vi "reportError.vi"(8 "ErrorIn":errorcluster, 10 "ErrorType":T1, 11 "QueuesIn":T2) -> (0 "ErrorOut":errorcluster, 3 "QueuesOut":T2)   [LabVIEW 2019]
uses:
  utilities/Queues.ctl
  UIVIs/UIInput.ctl
  UIVIs/UIOutput.ctl
  UIVIs/AccelerationDataFrames.ctl
  communicateWebServicesVIs/WebServicesData.ctl
  ErrorType.ctl
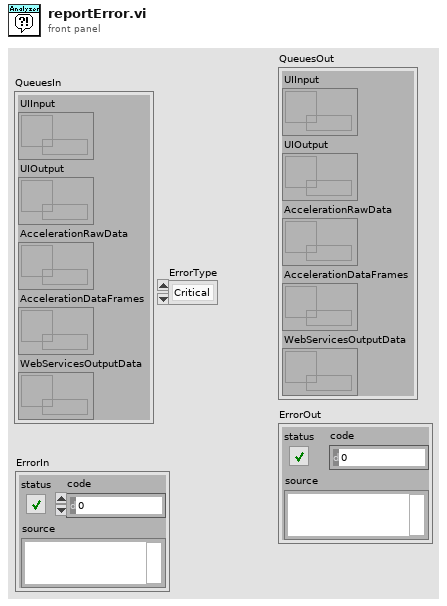
[diagram p1: front panel]
types:
  T1 = typedef "ErrorType.ctl" = enum16{"Critical", "Internal"}
  T2 = typedef "Queues.ctl" = cluster{"UIInput":refnum<queue>, "UIOutput":refnum<queue>, "AccelerationRawData":refnum<queue>, "AccelerationDataFrames":refnum<queue>, "WebServicesOutputData":refnum<queue>}
  T3 = typedef "UIOutput.ctl" = cluster{"Aquiring data":bool, "CriticalError":errorcluster, "InternalError":errorcluster, "FIFO overflow":bool, "Analyzing data":bool}
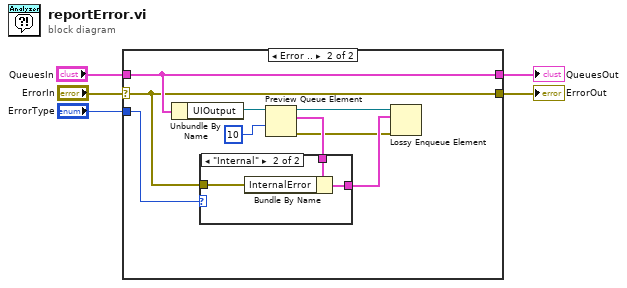
[diagram p0: block diagram]
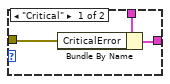
[diagram p3: hidden frame]
diagram:
  n1 = case shown="Error .." "ErrorIn" {
    selector: "ErrorIn" -> [w6 w9]
    tunnel: [w7 w13] -> w3
    tunnel: "QueuesIn" -> [w7 w13]
    tunnel: [w6 w9] -> w2
    tunnel: "ErrorType" -> [_ w12]
    frame No Error {
    }
    frame Error {
      n2 = Unbundle By Name(w13) -> ("UIOutput"=w16:refnum<queue>)
      n3 = Preview Queue Element(queue=w16, timeout in ms (-1)=10) -> (queue out=w14:refnum<queue>, element=w11:T3, error out=w8:errorcluster)  [unwired: 1 in, 1 out]
      n4 = case shown="\"Internal\"" w12 {
        tunnel: w11 -> [w19 w22]
        tunnel: [w18 w21] -> w10
        tunnel: w9 -> [w17 w20]
        frame "Critical" {
          n5 = Bundle By Name(cluster=w19, "CriticalError"=w17) -> (w18:T3)
        }
        frame "Internal" {
          n6 = Bundle By Name(cluster=w22, "InternalError"=w20) -> (w21:T3)
        }
      }
      n7 = Lossy Enqueue Element(queue=w14, element=w10, error in (no error)=w8) -> ()  [unwired: 4 out]
    }
  }
  "ErrorOut" <- w2
  "QueuesOut" <- w3
